vi "Create Folder if Needed.vi"(11 "Settings File Path":path) -> (3 "File Path Out":path=path "C:/Data/Settings.ini")   [LabVIEW 2019]
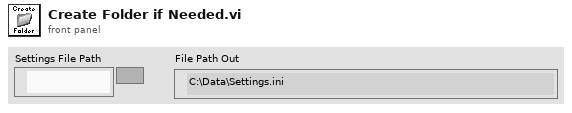
[diagram p1: front panel]
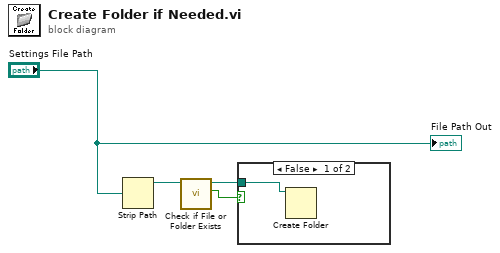
[diagram p0: block diagram]
diagram:
  n1 = Strip Path(path="Settings File Path") -> (stripped path=w2:path)  [unwired: 1 out]
  n2 = call <vilib>:"Check if File or Folder Exists.vi"("path"=w2) -> ("file or folder exists?"=w3:bool, "dup path"=w4:path)  [unwired: 8 in, 1 out]
  n3 = case shown="False" w3 {
    tunnel: w4 -> [w5 _]
    frame False {
      n4 = Create Folder(path (use dialog)=w5) -> ()  [unwired: 2 in, 3 out]
    }
    frame True {
    }
  }
  "File Path Out" <- "Settings File Path"
